vi "CameraSmallView.vi"(8 "XVerticalSlide 2":refnum<vi>, 9 "XHorizontalSlide 2":refnum<vi>, 10 "large cam ref":refnum<vi>, 11 "Big Camera":dbl[][](graph)) -> (3 "small cam view":dbl[][](array[numeric]))   [LabVIEW 2017]
uses:
  controls/xVerticalSlide/XVerticalSlide.xctl
  controls/xHorizontalSlide/XHorizontalSlide.xctl
panel:
  out "output cluster":T1
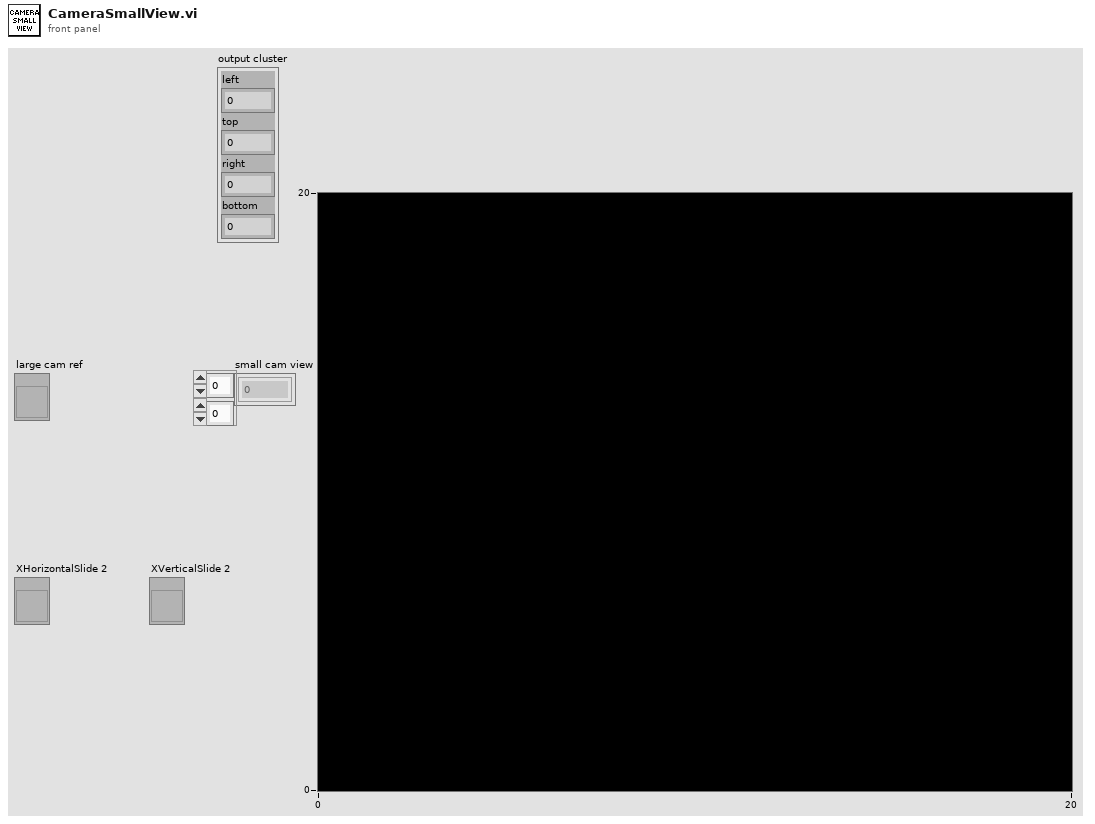
[diagram p1: front panel]
types:
  T1 = cluster{"left":i16, "top":i16, "right":i16, "bottom":i16}
  T2 = cluster{"[0]":i32, "[1]":i32, "[2]":i32, "[3]":i32, "[4]":i32, "[5]":i32, "[6]":i32, "[7]":i32, "[8]":i32}
  T3 = typedef "LVBoundsTypeDef.ctl" = cluster{"Width":u32, "Height":u32}
  T4 = cluster{"Width":i16, "Style":enum32{"Solid", "Dash", "Dot", "DashDot", "DashDotDot"}}
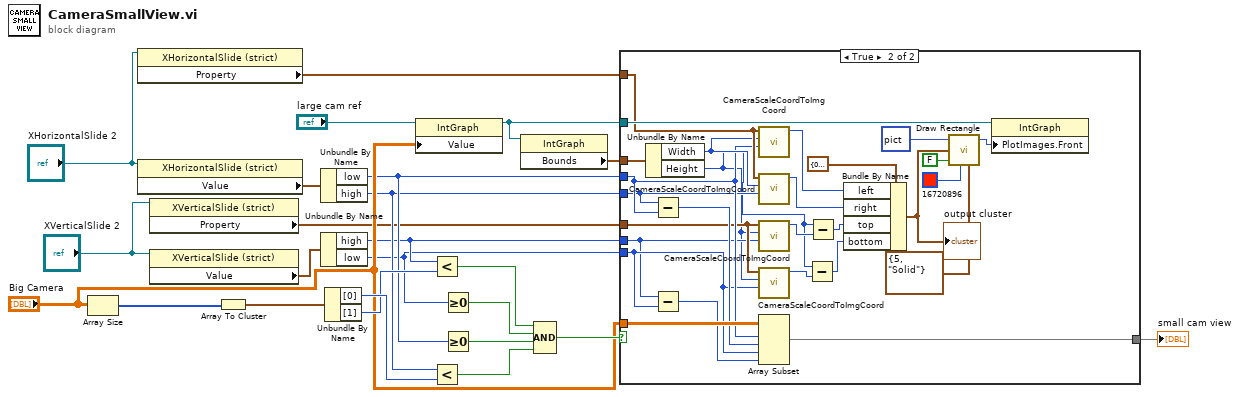
[diagram p0: block diagram]
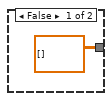
[diagram p2: hidden frame]
diagram:
  n1 = Array Size(array="Big Camera") -> (size(s)=w24:i32[])
  n2 = property class="XHorizontalSlide (strict)"(reference="XHorizontalSlide 2") -> ("Property"=w3:cluster{"min":i16, "max":i16})  [unwired: 1 in, 2 out]
  n3 = property class="XHorizontalSlide (strict)"(reference="XHorizontalSlide 2") -> ("Value"=w11:cluster{"low":i16, "high":i16})  [unwired: 1 in, 2 out]
  n4 = property class="XVerticalSlide (strict)"(reference="XVerticalSlide 2") -> ("Property"=w1:cluster{"min":i16, "max":i16})  [unwired: 1 in, 2 out]
  n5 = property class="XVerticalSlide (strict)"(reference="XVerticalSlide 2") -> ("Value"=w8:cluster{"low":i16, "high":i16})  [unwired: 1 in, 2 out]
  n6 = Array To Cluster(array=w24) -> (cluster=w23:T2)
  n7 = Unbundle By Name(w11) -> ("low"=w10:i16, "high"=w9:i16)
  n8 = Unbundle By Name(w8) -> ("high"=w7:i16, "low"=w6:i16)
  n9 = Unbundle By Name(w23) -> ("[0]"=w22:i32, "[1]"=w21:i32)
  n10 = property class="IntGraph"(reference="large cam ref", "Value"="Big Camera") -> (reference out=w12:refnum<vi>)  [unwired: 1 in, 1 out]
  n11 = Less?(x=w7, y=w21) -> (x < y?=w20:bool)
  n12 = Less?(x=w9, y=w22) -> (x < y?=w17:bool)
  n13 = Greater Or Equal To 0?(x=w6) -> (x >= 0?=w19:bool)
  n14 = Greater Or Equal To 0?(x=w10) -> (x >= 0?=w18:bool)
  n15 = property class="IntGraph"(reference=w12) -> ("Bounds"=w4:T3)  [unwired: 1 in, 2 out]
  n16 = Compound Arithmetic op=AND(w20, w19, w18, w17) -> (w16:bool)
  n17 = case shown="True" w16 {
    tunnel: "Big Camera" -> [_ w52]
    tunnel: w10 -> [_ w36]
    tunnel: w7 -> [_ w32]
    tunnel: w6 -> [_ w33]
    tunnel: [dbl[][] [] w49] -> w15
    tunnel: w9 -> [_ w35]
    tunnel: w12 -> [_ w44]
    tunnel: w4 -> [_ w43]
    tunnel: w3 -> [_ w40]
    tunnel: w1 -> [_ w34]
    frame False {
    }
    frame True {
      n18 = Unbundle By Name(w43) -> ("Width"=w37:u32, "Height"=w26:u32)
      n19 = Subtract(x=w35, y=w36) -> (x-y=w50:i16)
      n20 = Subtract(x=w32, y=w33) -> (x-y=w51:i16)
      n21 = call "CameraScaleCoordToImgCoord.vi"("value"=w36, "img size"=w37, "scale bounds"=w40) -> ("coord out"=w39:i32)  [unwired: 8 in]
      n22 = call "CameraScaleCoordToImgCoord.vi"("value"=w35, "img size"=w37, "scale bounds"=w40) -> ("coord out"=w38:i32)  [unwired: 8 in]
      n23 = call "CameraScaleCoordToImgCoord.vi"("value"=w32, "img size"=w26, "scale bounds"=w34) -> ("coord out"=w27:i32)  [unwired: 8 in]
      n24 = call "CameraScaleCoordToImgCoord.vi"("value"=w33, "img size"=w26, "scale bounds"=w34) -> ("coord out"=w28:i32)  [unwired: 8 in]
      n25 = Array Subset(array=w52, index (row)=w36, length (row)=w50, index (col)=w33, length (col)=w51) -> (w49:dbl[][])
      n26 = Subtract(x=w26, y=w28) -> (x-y=w29:u32)
      n27 = Subtract(x=w26, y=w27) -> (x-y=w30:u32)
      n28 = Bundle By Name(cluster=T1 {"left"=0, "top"=0, "right"=0, "bottom"=0} ("rect"), "left"=w39, "right"=w38, "top"=w30, "bottom"=w29) -> (w42:T1)
      "output cluster" <- w42
      n29 = call <vilib>:"Draw Rectangle.vi"("picture"=picture data[5B], "rect"=w42, "fill?(F)"=FALSE, "color(black)"=u32 16720896, "pen"=T4 {"Width"=5, "Style"=enum."Solid"}) -> ("new picture"=w45:picture)  [unwired: 4 in]
      n30 = property on="Property Node" class="IntGraph"(reference=w44, "PlotImages.Front"=w45) -> ()  [unwired: 1 in, 2 out]
    }
  }
  "small cam view" <- w15
